vi "clean_raw_data_every2.vi"(8 "error in (no error)":errorcluster, 9 "data raw":cluster{"I":i32[][], "II":i32[][]}, 10 "N of scans":i32, 11 "VIS-NIR_STRESING_NEW in":refnum<class "VIS-NIR_STRESING_NEW.lvclass">) -> (0 "error out":errorcluster, 1 "I 2":i32[][](array[numeric]), 2 "I":i32[][](array[numeric]), 3 "VIS-NIR_STRESING_NEW out":refnum<class "VIS-NIR_STRESING_NEW.lvclass">)   [LabVIEW 2020, in "VIS-NIR_STRESING_NEW.lvclass"]
uses:
  VIS-NIR_STRESING_NEW.lvclass
panel:
  in  "exchange I and II":bool
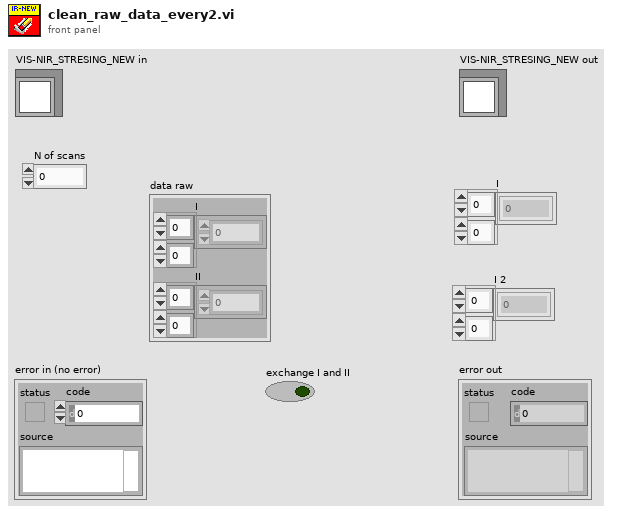
[diagram p1: front panel]
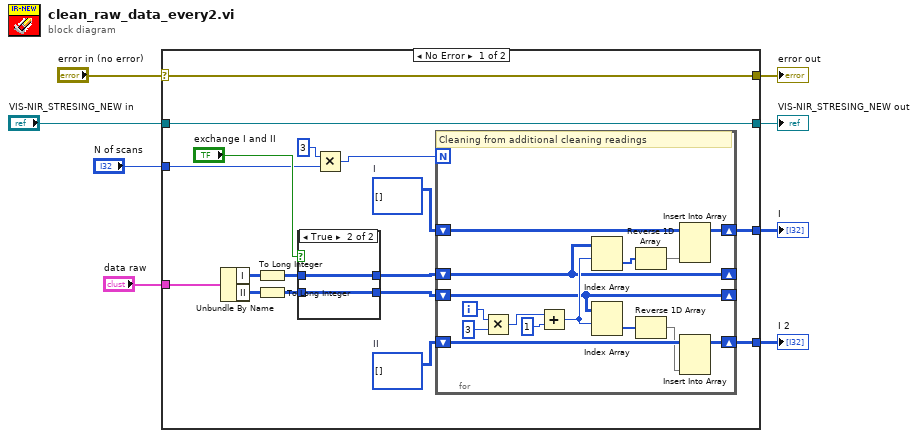
[diagram p0: block diagram]
diagram:
  n1 = case shown="No Error" "error in (no error)" {
    selector: "error in (no error)" -> [w17 w46]
    tunnel: [w17 w46] -> w4
    tunnel: [w25 w45] -> w6
    tunnel: "VIS-NIR_STRESING_NEW in" -> [w25 w45]
    tunnel: [w16 _] -> w3
    tunnel: [w15 _] -> w2
    tunnel: "N of scans" -> [w14 _]
    tunnel: "data raw" -> [w13 _]
    frame No Error {
      w24 = i32[][] []  # II
      w23 = i32[][] []  # I
      n2 = Unbundle By Name(w13) -> ("I"=w12:i32[][], "II"=w11:i32[][])
      n3 = To Long Integer(number=w12) -> (32bit integer=w21:i32[][])
      n4 = To Long Integer(number=w11) -> (32bit integer=w22:i32[][])
      n5 = case shown="True" "exchange I and II" {
        tunnel: [w41 w44] -> w19
        tunnel: w21 -> [w42 w44]
        tunnel: w22 -> [w41 w43]
        tunnel: [w42 w43] -> w20
        frame False {
        }
        frame True {
        }
      }
      n6 = Multiply(x=3, y=w14) -> (x*y=w10:i32)
      n7 = for {
        N: w10 -> [_]
        shift-right: [w31] -> _
        shift-left: w19 -> [w31]
        shift-right: [w30] -> _
        shift-left: w20 -> [w30]
        shift-right: [w39] -> w16
        shift-left: w23 -> [w40]
        shift-right: [w38] -> w15
        shift-left: w24 -> [w37]
        i -> [w36]
        # "Cleaning from additional cleaning readings"
        n8 = Multiply(x=w36, y=3) -> (x*y=w34:i32)
        n9 = Add(x=w34, y=1) -> (x+y=w32:i32)
        n10 = Index Array(array=w31, index (row)=w32) -> (element=w27:i32[])  [unwired: 1 in]
        n11 = Index Array(array=w30, index (row)=w32) -> (element=w29:i32[])  [unwired: 1 in]
        n12 = Reverse 1D Array(array=w27) -> (reversed array=w26:i32[])
        n13 = Reverse 1D Array(array=w29) -> (reversed array=w28:i32[])
        n14 = Insert Into Array(array=w40, new element=w26) -> (w39:i32[][])  [unwired: 2 in]
        n15 = Insert Into Array(array=w37, new element=w28) -> (w38:i32[][])  [unwired: 2 in]
      }
    }
    frame Error {
    }
  }
  "error out" <- w4
  "VIS-NIR_STRESING_NEW out" <- w6
  "I" <- w3
  "I 2" <- w2
